vi "KeyControl.vi"() -> ()   [LabVIEW 2010]
uses:
  <vilib>/userDefined/High Color/IMAQdx.ctl
  BotCommands.ctl
  <vilib>/Platform/TimedLoop/XDataNode/XDataNode.xnode
  <vilib>/Platform/TimedLoop/XDataNode/timing_clust.ctl
  <vilib>/Platform/TimedLoop/XDataNode/nitl_modes.ctl
  <vilib>/Platform/TimedLoop/XDataNode/wakeup.ctl
  <vilib>/Utility/inputDevices.llb/closeJoystick.vi
  <vilib>/Utility/inputDevices.llb/joystickAcquire.vi
  <vilib>/Platform/TimedLoop/XDataNode/XDNodeRunTimeDep.lvlib
  <vilib>/vision/driver/NI_Vision_Acquisition_Software.lvlib
panel:
  in  "Target Address":string="10.25.1.100"
  out "?":T1(plugin-control)
  in  "Camera Name":T2="cam0"
  out "Image Error":errorcluster
  out "Rotation":dbl(knob) scale=1.0..-1.0
  out "Speed":dbl(knob) scale=-1.0..1.0
  in  "Turn scale":dbl=0.7
  in  "Speed scale":dbl=0.5
  out "Control Error":errorcluster
  in  "stop":bool
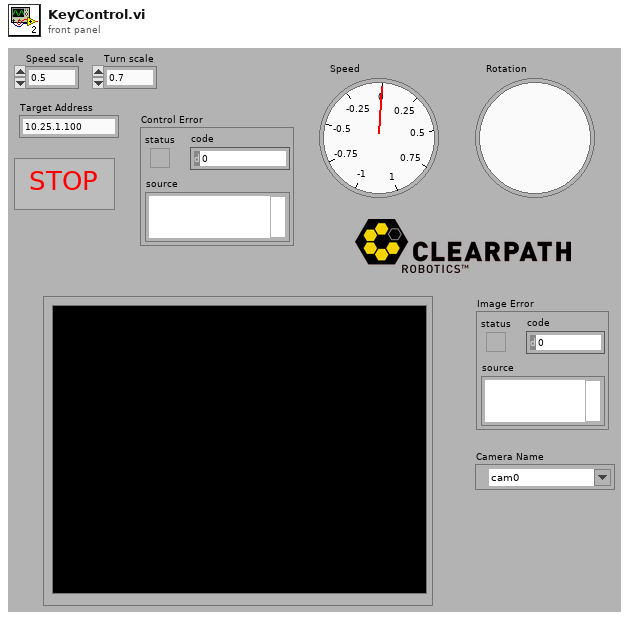
[diagram p1: front panel]
types:
  T1 = typedef "IMAQ Image.ctl" = refnum<image>
  T2 = typedef "IMAQdx.ctl" = refnum<k21>
  T3 = typedef "BotCommands.ctl" = cluster{"Translational":dbl, "Rotational":dbl}
  T4 = typedef "XDNodeRunTimeDep.lvlib/timing_clust.ctl" = cluster{"Expected End [f-1]":u64, "Actual End [f-1]":u64, "Finished Late? [f-1]":bool, "Expected End [i-1]":u64, "Actual End [i-1]":u64, "Finished Late? [i-1]":bool, "Expected Start [i]":u64, "Actual Start [i]":u64, "Expected Start [f]":u64, "Actual Start [f]":u64, "Source Name":string, "Structure Name":string, "Period":i64, "Deadline":i64, "Offset":i64, "Start":i64, "Priority":i32, "Timeout":i32, "Mode":T5, "Wakeup Reason":T6, "Error":errorcluster, "Source Type":string, "Secondary Source Type":string, "Global End Time":u64, "Global Start Time":u64, "Frame Duration":u64, "Iteration Duration":u64, "Assigned CPU":i32, "I/O Scan Engine Mode":u32}
  T5 = typedef "XDNodeRunTimeDep.lvlib/nitl_modes.ctl" = enum32{"No Change", "Process missed periods, maintain original phase", "Discard missed periods, maintain original phase", "Process missed periods, ignore original phase", "Discard missed periods, ignore original phase"}
  T6 = typedef "XDNodeRunTimeDep.lvlib/wakeup.ctl" = enum32{"Normal", "Aborted", "Asynchronous wakeup", "Timing source error", "Timed loop error", "Timeout"}
  T7 = cluster{"X axis":i32, "Y axis":i32, "Z axis":i32, "X axis rotation":i32, "Y axis rotation":i32, "Z axis rotation":i32, "U axis":i32, "V axis":i32}
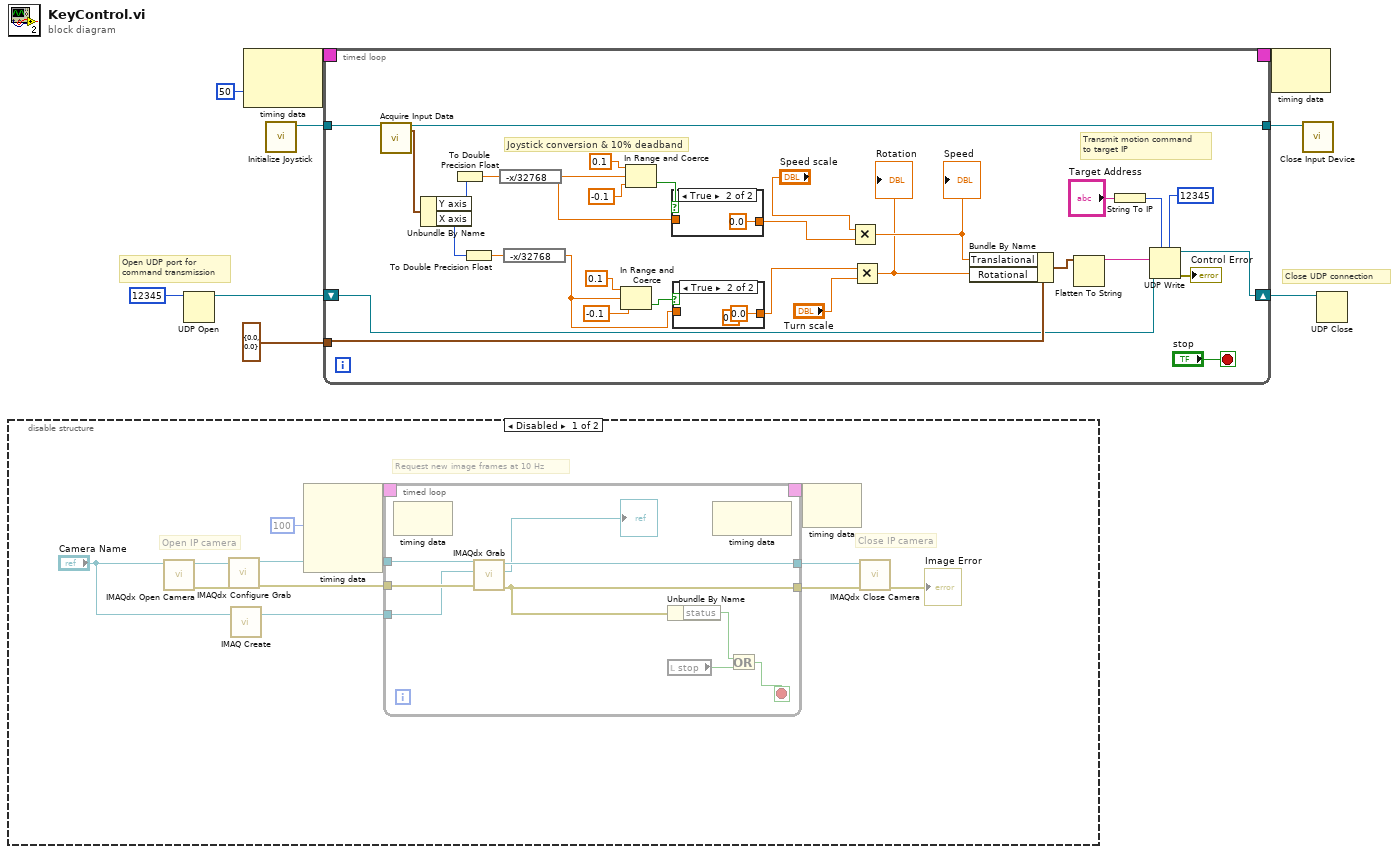
[diagram p0: block diagram]
diagram:
  # "Close UDP connection"
  # "Open UDP port for\ncommand transmission"
  n1 = disable-structure shown="Disabled" {
    frame Disabled {
      # "Request new image frames at 10 Hz"
      # "Close IP camera"
      # "Open IP camera"
      n2 = call <vilib>:"IMAQdx Open Camera.vi"("Session In"="Camera Name") -> ("error out"=w18:errorcluster, "Session Out"=w19:T2)  [unwired: 9 in]
      n3 = call <vilib>:"IMAQdx Configure Grab.vi"("error in"=w18, "Session In"=w19) -> ("error out"=w16:errorcluster, "Session Out"=w17:T2)  [unwired: 8 in]
      n4 = call "IMAQ Create"("Image Name"="Camera Name") -> ("New Image"=w15:T1)  [unwired: 4 in, 1 out]
      n5 = node-c288(i64 100 ("Period")) -> (w21:T4)  [unwired: 3 in]
      n6 = timed-loop {
        tunnel: w17 -> [w30]
        tunnel: w16 -> [w29]
        tunnel: w15 -> [w28]
        tunnel: [w24] -> w14
        tunnel: [w27] -> w12
        timing: w21 -> [_]
        timing-out: [_] -> w20
        stop <- w25 stop-if-true
        n7 = node-c288() -> ()  [unwired: 1 in, 1 out]
        n8 = call <vilib>:"IMAQdx Grab.vi"("error in"=w29, "Image In"=w28, "Session In"=w30) -> ("error out"=w24:errorcluster, "Image Out"=→"?":T1, "Session Out"=w27:T2)  [unwired: 5 in, 1 out]
        n9 = Unbundle By Name(w24) -> ("status"=w26:bool)
        n10 = local read "stop"() -> (w22:bool)
        n11 = node-c288() -> ()  [unwired: 1 in, 1 out]
        n12 = Or(x=w26, y=w22) -> (x .or. y?=w25:bool)
      }
      n13 = node-c288(w20) -> ()  [unwired: 1 out]
      n14 = call <vilib>:"IMAQdx Close Camera.vi"("error in"=w14, "Session In"=w12) -> ("error out"=→"Image Error":errorcluster)  [unwired: 9 in]
    }
    frame Enabled {
    }
  }
  n15 = UDP Open(11:u16 12345 ("remote port")) -> (port=w1:refnum<k16>)  [unwired: 4 in, 2 out]
  n16 = node-c288(i64 50 ("Period")) -> (w9:T4)  [unwired: 1 in]
  n17 = call <vilib>:"Initialize Joystick.vi"() -> ("device ID"=w3:refnum<k1>)  [unwired: 10 in, 1 out]
  n18 = timed-loop {
    tunnel: w3 -> [w66]
    tunnel: [w65] -> w7
    tunnel: T3 {"Translational"=0.0, "Rotational"=0.0} ("BotCommands") -> [w64]
    shift-right: [w44] -> w5
    shift-left: w1 -> [w47]
    timing: w9 -> [_]
    timing-out: [_] -> w8
    stop <- "stop" stop-if-true
    (unwired) 0.0
    # "Joystick conversion & 10% deadband"
    # "Transmit motion command \nto target IP"
    n19 = call-poly <vilib>:"Acquire Input Data.vi"("device ID"=w66) -> ("device ID"=w65:refnum<k1>, "axis info"=w62:T7)  [unwired: 14 in, 3 out]
    n20 = Unbundle By Name(w62) -> ("Y axis"=w61:i32, "X axis"=w60:i32)
    n21 = To Double Precision Float(number=w61) -> (double precision float=w59:dbl)
    n22 = To Double Precision Float(number=w60) -> (double precision float=w58:dbl)
    n23 = expression code="-x/32768"(w59) -> (w52:dbl)
    n24 = expression code="-x/32768"(w58) -> (w48:dbl)
    n25 = In Range and Coerce(upper limit=0.1, x=w48, lower limit=-0.1 ("upper limit")) -> (In Range?=w49:bool)  [unwired: 1 out]
    n26 = In Range and Coerce(upper limit=0.1, x=w52, lower limit=-0.1 ("upper limit")) -> (In Range?=w55:bool)  [unwired: 1 out]
    n27 = case shown="True" w55 {
      tunnel: [w70 0.0] -> w39
      tunnel: w52 -> [w70 _]
      frame False {
      }
      frame True {
      }
    }
    n28 = case shown="True" w49 {
      tunnel: [w68 0.0] -> w38
      tunnel: w48 -> [w68 _]
      frame False {
      }
      frame True {
      }
    }
    n29 = Multiply(x="Speed scale", y=w39) -> (x*y=w57:dbl)
    "Speed" <- w57
    n30 = Multiply(x=w38, y="Turn scale") -> (x*y=w56:dbl)
    "Rotation" <- w56
    n31 = Bundle By Name(cluster=w64, "Translational"=w57, "Rotational"=w56) -> (w63:T3)
    n32 = Flatten To String(anything=w63) -> (data string=w46:string)  [unwired: 2 in, 3 out]
    n33 = String To IP(1:"Target Address") -> (0:w42:u32)
    n34 = UDP Write(address=w42, port or service name=u16 12345, connection ID=w47, data in=w46) -> (error out=→"Control Error":errorcluster, 3:w44:refnum<k16>)  [unwired: 2 in]
  }
  n35 = node-c288(w8) -> ()  [unwired: 1 out]
  n36 = call-poly <vilib>:"Close Input Device.vi"("device ID"=w7) -> ()  [unwired: 9 in, 1 out]
  n37 = UDP Close(connection ID=w5) -> ()  [unwired: 1 in, 2 out]
